vi "Destroy User Event - Stop.vi"(8 "error in (no error)":cluster{"状态":bool, "代码":i32, "源":string} caption="错误输入（无错误）", 11 "用户事件－停止":refnum<user-event>) -> (0 "error out":cluster{"状态":bool, "代码":i32, "源":string} caption="错误输出")   [LabVIEW 2022 SP3, in "User Event - Stop.lvlib"]
doc: "无论是否即将出错，销毁用户事件。"
uses:
  User Event - Stop.lvlib
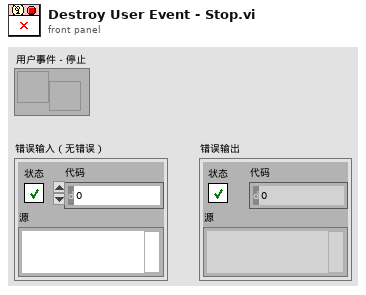
[diagram p1: front panel]
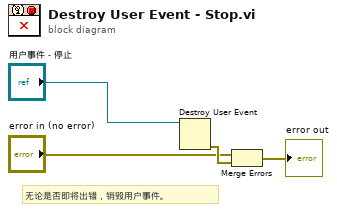
[diagram p0: block diagram]
diagram:
  # "无论是否即将出错，销毁用户事件。"
  n1 = Destroy User Event(user event="用户事件－停止") -> (error out=w3:errorcluster)  [unwired: 1 in]
  n2 = Merge Errors("error in (no error)", w3) -> (→"error out":errorcluster)
